vi "Set pin command.vi"(0 "Serial Device in":refnum<class "Serial Device.lvclass">, 1 "Puerto":string(combo), 2 "Pin":string(combo), 3 "Valor":string(combo), 5 "error in (no error)":errorcluster, 6 "Marca":string) -> (14 "Serial Device out":refnum<class "Serial Device.lvclass">, 15 "Command":string, 17 "Expected response":string, 19 "error out":errorcluster)   [LabVIEW 2020, in "Serial Device.lvclass"]
doc: "Aqui se forma el comando para poner el pin de un puerto en alto o bajo, y dependiendo de la marca que se le coloque."
uses:
  Serial Device.lvclass
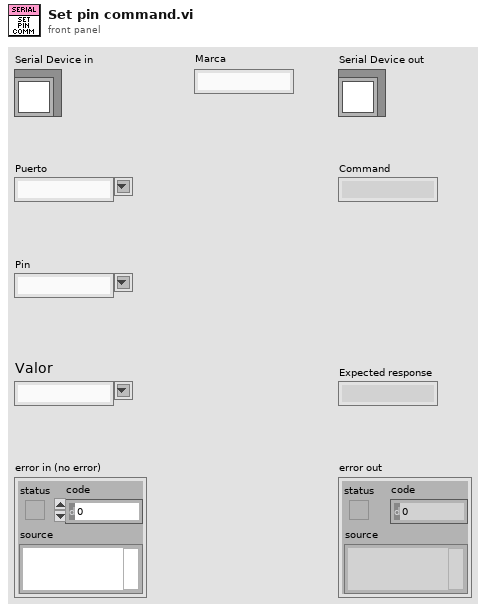
[diagram p1: front panel]
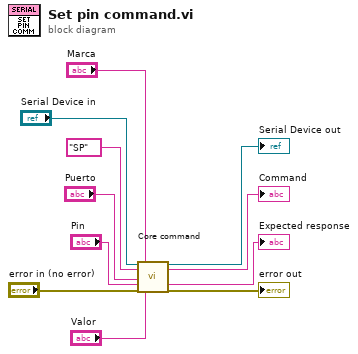
[diagram p0: block diagram]
diagram:
  n1 = call-dynamic "Core command.vi"("object in"="Serial Device in", "Command"="SP", "Param1"="Puerto", "Param2"="Pin", "error in (no error)"="error in (no error)", "Marca"="Marca", "Param3"="Valor") -> ("object out"=→"Serial Device out":refnum<class "Serial Device.lvclass">, "Command"=→"Command":string, "Expected response"=→"Expected response":string, "error out"=→"error out":errorcluster)  [unwired: 9 in]
